vi "Stop Command.vi"() -> (2 "Stop":string)   [LabVIEW 2017]
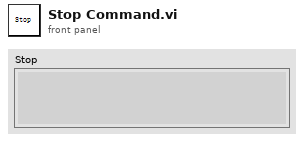
[diagram p1: front panel]
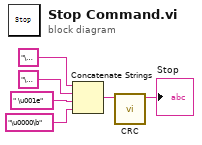
[diagram p0: block diagram]
diagram:
  n1 = Concatenate Strings("\u0001", "\u0006", " \u001e", "\u0000\b") -> (w2:string)
  n2 = call "CRC.vi"("字符串"=w2) -> ("连接的字符串"=→"Stop":string)  [unwired: 9 in, 1 out]
